vi "Main.vi"() -> ()   [LabVIEW 2021]
uses:
  Sub VIs/Trajectory Control/Trajectory_Control.ctl
  Sub VIs/Logging/Controller Data.ctl
  Sub VIs/Drive Motor/Drive Motor Data.ctl
  Sub VIs/Steering Motor/Steering Motor Data.ctl
  Sub VIs/State Estimator/State Estimate.ctl
  Sub VIs/State Estimator/Measurements.ctl
  Sub VIs/IMU/IMU Data.ctl
  Sub VIs/Steering Motor Encoder/Steering Motor Encoder Data.ctl
  Sub VIs/GNSS/GNSS Data.ctl
  <vilib>/Utility/RT CPU Load.ctl
  Sub VIs/Logging/Log Level.ctl
  <vilib>/Platform/TimedLoop/XDataNode/timing_clust.ctl
  <vilib>/Platform/TimedLoop/XDataNode/nitl_modes.ctl
  <vilib>/Platform/TimedLoop/XDataNode/wakeup.ctl
  Sub VIs/Steering Motor/Steering Motor Handle.ctl
  <vilib>/platform/TimedLoop/XDataNode/XDataNode.xnode
  <vilib>/Platform/TimedLoop/XDataNode/XDNodeRunTimeDep.lvlib
  <vilib>/NI_Real-Time Target Support.lvlib
panel:
  in  "Set Speed / Set Current\n(Built-in)  /  (PI Controller)":bool
  in  "Current at Steady State":dbl=5.5
  in  "Threshold":dbl=0.5
  out "?":bool
  in  "Open Loop Current Flag":bool
  in  "Open Loop Current":dbl min=0.0
  out "Abort Trajectory Enabled":bool
  out "Roll angle (rad)":dbl(graph)
  out "Indoor Enabled 2":bool
  in  "Indoor (RollRef)":bool
  out "Indoor Enabled":bool
  in  "Indoor (NoGPS)":bool
  out "Input and Motor Current (A)":T1(graph)
  out "Gyroscope (rad/s)":T2(graph)
  in  "No Kf":bool
  out "No Kf flag":bool
  in  "Kf":dbl
  in  "Abort Trajectory":bool
  in  "Kp":dbl
  in  "Ki":dbl
  out "Speed":bool
  in  "?":bool
  out "RPM":bool
  in  "Drive Motor Ref Speed (m/s)":dbl
  in  "file path (trajectorymat)":path=path "c:/ni-rt/startup/trajectorymat_parking_line.csv"
  in  "file path (matrixmat)":path=path "c:/ni-rt/startup/matrixmat_default.csv"
  out "velocity":dbl(graph)
  out "CPU loads":T3[](array[typedef]) {"ISR (%)" format="%#.2f"; "Idle (%)" format="%#.2f"; "Background (%)" format="%#.2f"; "Normal (%)" format="%#.2f"; "Above Normal (%)" format="%#.2f"; "High (%)" format="%#.2g"; "Timed Structures (%)" format="%#.2g"; "Time Critical (%)" format="%#.2g"; "Total (%)" format="%#.2g"}
  out "Measurements (Debug)":T4 {"GNSS Data"."Longitude (deg)" format="%#.10g"; "GNSS Data"."Latitude (deg)" format="%#.10g"; "GNSS Data"."Longitude (rad)" format="%#_10g"; "GNSS Data"."Latitude (rad)" format="%#_10g"}
  out "State Estimate (Debug)":T8 {"Y (m)" format="%#_10g"; "X (m)" format="%#_10g"}
  out "Motor Controllers (Debug)":T9
  out "Trajectory (Debug)":T12
  out "State estimator Ts check":bool
  out "E2 limit hit":bool
  out "E1 limit hit":bool
  out "XY trajectory (0 is bikeposition)":T13(graph)
  out "Y-Offset":dbl
  out "X-Offset":dbl
  in  "Reset and Init trajectory":bool
  in  "Drive Motor Ref Angular Speed (rad/s)":dbl
  in  "Enable Steering Motor":bool
  out "Steering Motor Enabled":bool
  out "Abort":bool
  in  "Reset Steering Motor Encoder":bool
  in  "Stop Button":bool
  # "To be set before running"
  # "PI Speed Controller"
  # "Scooter: \nKi=0.1, Kp=0.3\nGreen bike:\nKi=0.5, Kp=1.4\nRed bike\nKi=0.2, Kp=1.5"
  # "RED bike roller: 2.5\nGREEN bike roller: 5.5\nGREEN bike outside: 4.4"
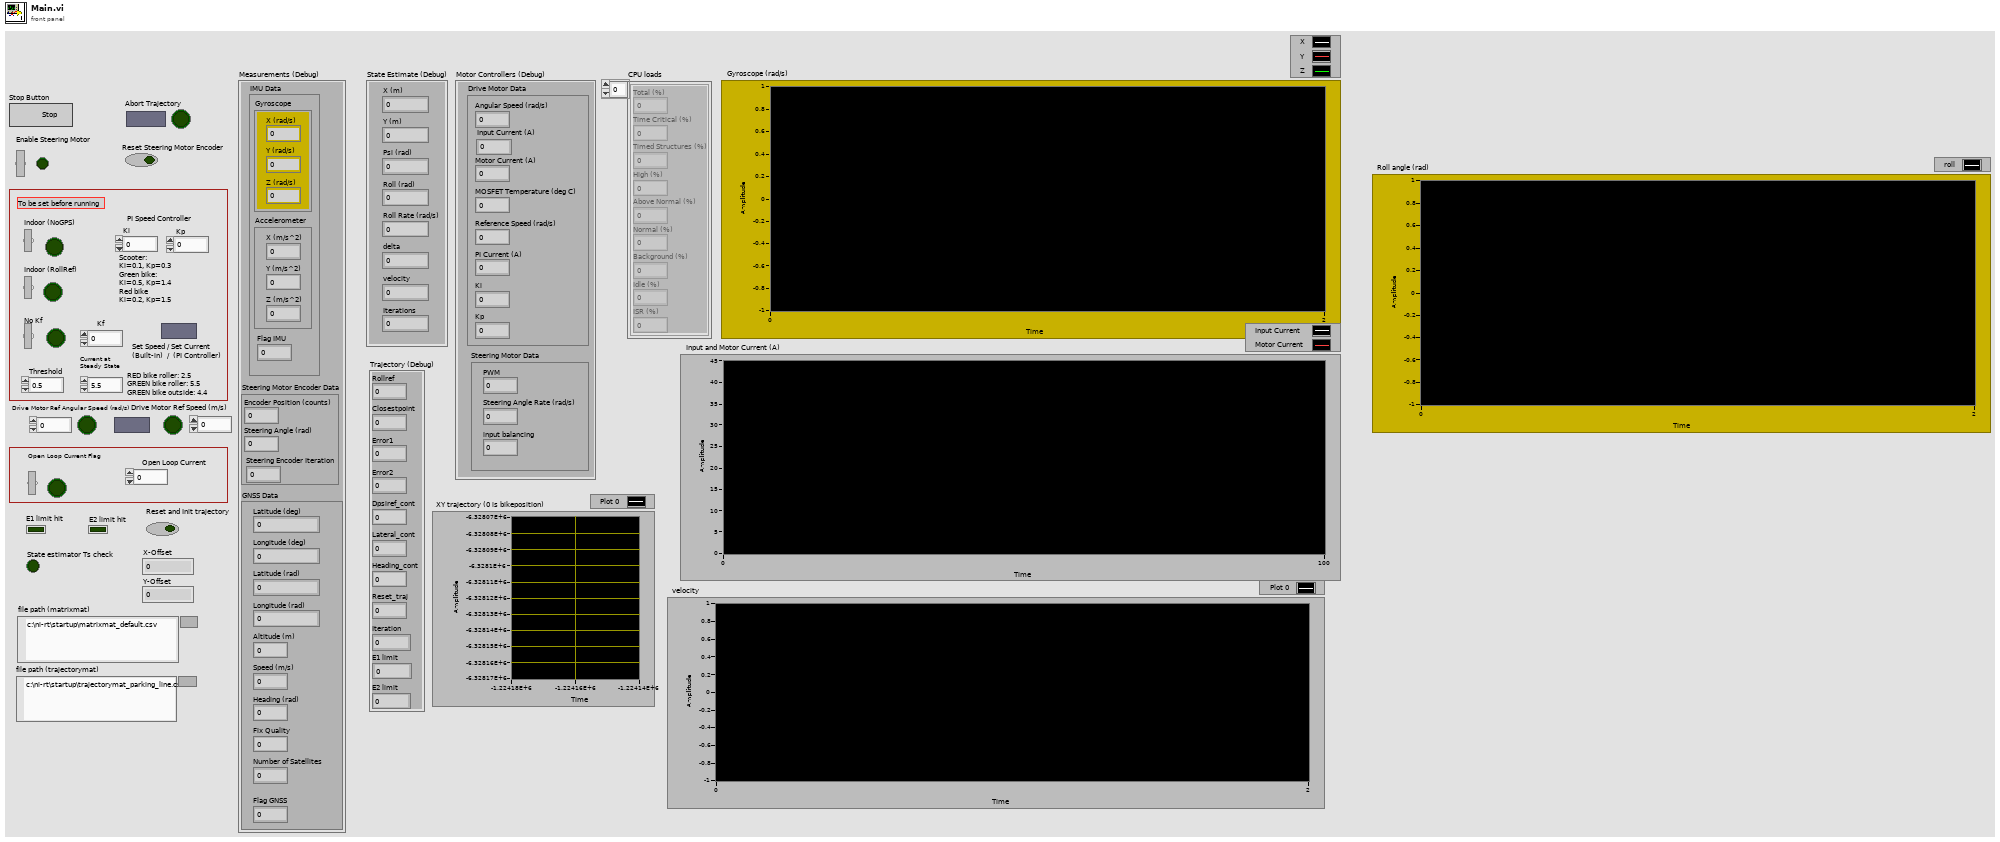
[diagram p1: front panel]
types:
  T1 = cluster{"Input Current (A)":dbl, "Motor Current (A)":dbl}
  T2 = cluster{"X (rad/s)":dbl, "Y (rad/s)":dbl, "Z (rad/s)":dbl}
  T3 = typedef "NI_Real-Time Target Support.lvlib/RT CPU Load.ctl" = cluster{"Total (%)":dbl, "Time Critical (%)":dbl, "Timed Structures (%)":dbl, "High (%)":dbl, "Above Normal (%)":dbl, "Normal (%)":dbl, "Background (%)":dbl, "Idle (%)":dbl, "ISR (%)":dbl}
  T4 = typedef "Measurements.ctl" = cluster{"IMU Data":T5, "Steering Motor Encoder Data":T6, "GNSS Data":T7}
  T5 = typedef "IMU Data.ctl" = cluster{"Gyroscope":cluster{"X (rad/s)":dbl, "Y (rad/s)":dbl, "Z (rad/s)":dbl}, "Accelerometer":cluster{"X (m/s^2)":dbl, "Y (m/s^2)":dbl, "Z (m/s^2)":dbl}, "Flag IMU":dbl}
  T6 = typedef "Steering Motor Encoder Data.ctl" = cluster{"Encoder Position (counts)":i32, "Steering Angle (rad)":dbl, "Steering Encoder Iteration":dbl}
  T7 = typedef "GNSS Data.ctl" = cluster{"Latitude (rad)":dbl, "Longitude (rad)":dbl, "Altitude (m)":dbl, "Speed (m/s)":dbl, "Heading (rad)":dbl, "Fix Quality":i32, "Number of Satellites":i32, "Latitude (deg)":dbl, "Longitude (deg)":dbl, "Flag GNSS":dbl}
  T8 = typedef "State Estimate.ctl" = cluster{"X (m)":dbl, "Y (m)":dbl, "Psi (rad)":dbl, "Roll (rad)":dbl, "Roll Rate (rad/s)":dbl, "delta":dbl, "velocity":dbl, "Iterations":dbl}
  T9 = typedef "Controller Data.ctl" = cluster{"Drive Motor Data":T10, "Steering Motor Data":T11}
  T10 = typedef "Drive Motor Data.ctl" = cluster{"Angular Speed (rad/s)":dbl, "Input Current (A)":dbl, "Motor Current (A)":dbl, "MOSFET Temperature (deg C)":dbl, "Reference Speed (rad/s)":dbl, "PI Current (A)":dbl, "Ki":dbl, "Kp":dbl}
  T11 = typedef "Steering Motor Data.ctl" = cluster{"PWM":dbl, "Steering Angle Rate (rad/s)":dbl, "input balancing":dbl}
  T12 = typedef "Trajectory_Control.ctl" = cluster{"Rollref":dbl, "Closestpoint":dbl, "Error1":dbl, "Error2":dbl, "Dpsiref_cont":dbl, "Lateral_cont":dbl, "Heading_cont":dbl, "Reset_traj":dbl, "Iteration":dbl, "E1 limit":u32, "E2 limit":u32}
  T13 = cluster{"Trajectory(X/Y/PSI)":dbl[], "Trajectory(X/Y/PSI)":dbl[]}
  T14 = cluster{"Steering Angle Rate":dbl, "rollReference":dbl, "roll":dbl, "rollRate":dbl, "Kp":dbl, "Kd":dbl, "steering_flag":i32}
  T15 = typedef "XDNodeRunTimeDep.lvlib/timing_clust.ctl" = cluster{"Expected End [f-1]":u64, "Actual End [f-1]":u64, "Finished Late? [f-1]":bool, "Expected End [i-1]":u64, "Actual End [i-1]":u64, "Finished Late? [i-1]":bool, "Expected Start [i]":u64, "Actual Start [i]":u64, "Expected Start [f]":u64, "Actual Start [f]":u64, "Source Name":string, "Structure Name":string, "Period":i64, "Deadline":i64, "Offset":i64, "Start":i64, "Priority":i32, "Timeout":i32, "Mode":T16, "Wakeup Reason":T17, "Error":errorcluster, "Source Type":string, "Secondary Source Type":string, "Global End Time":u64, "Global Start Time":u64, "Frame Duration":u64, "Iteration Duration":u64, "Assigned CPU":i32, "I/O Scan Engine Mode":u32}
  T16 = typedef "XDNodeRunTimeDep.lvlib/nitl_modes.ctl" = enum32{"No Change", "Process missed periods, maintain original phase", "Discard missed periods, maintain original phase", "Process missed periods, ignore original phase", "Discard missed periods, ignore original phase"}
  T17 = typedef "XDNodeRunTimeDep.lvlib/wakeup.ctl" = enum32{"Normal", "Aborted", "Asynchronous wakeup", "Timing source error", "Timed loop error", "Timeout"}
  T18 = typedef "Steering Motor Handle.ctl" = cluster{"Dummy":dbl}
  T19 = typedef "Log Level.ctl" = enum16{"Error", "Warning", "Info"}
  T20 = cluster{"B":dbl[], "A":dbl[][], "C":dbl[][], "D":dbl[], "K":dbl[][], "Trajectory":dbl[][], "Init":dbl[], "parameter":dbl[][], "K_noGPS":dbl[][]}
  T21 = typedef "Configuration.ctl" = cluster{"Accelerometer Bias":cluster{"X (m/s)":dbl, "Y (m/s)":dbl, "Z (m/s)":dbl}, "Gyroscope Bias":cluster{"X (m/s)":dbl, "Y (m/s)":dbl, "Z (m/s)":dbl}, "Steering Motor Gear Ratio":dbl, "Steering Pully Gear Ratio":dbl, "Steering Encoder CPR":dbl, "Steering Motor Max RPM":dbl, "Wheelbase (m)":dbl, "Fork Angle (rad)":dbl, "Balancing Controller":cluster{"Kp (/s)":dbl, "Kd (1)":dbl}, "Max Allowed Steering Angle (rad)":dbl, "Task Periods":cluster{"Emergency Stop (us)":i64, "IMU (us)":i64, "Steering Motor Encoder (us)":i64, "State Estimator (us)":i64, "Balancing Controller (us)":i64, "GNSS (us)":i64, "Logging (us)":i64, "Drive Motor (us)":i64, "Visualization (us)":i64}, "Drive Motor Gear Ratio":dbl, "lr":dbl, "lf":dbl, "lambda":dbl, "k1":dbl, "k2":dbl, "e1_max":dbl, "Ad_t":dbl, "Bd_t":dbl, "C_t":dbl, "D_t":dbl, "Wheel radius":dbl}
  T22 = typedef "NI_Matrix.lvlib/RealMatrix.ctl" = dbl[][]
  T23 = typedef "GNSS Handle.ctl" = cluster{"VISA Resource Name":refnum<visa-resource-name>}
  T24 = typedef "IMU Handle.ctl" = cluster{"I2C address":u8}
  T25 = typedef "Drive Motor Handle.ctl" = cluster{"VISA Resource Name":refnum<visa-resource-name>}
  T26 = typedef "Log Handle.ctl" = cluster{"Data File":refnum<file>, "Event File":refnum<file>}
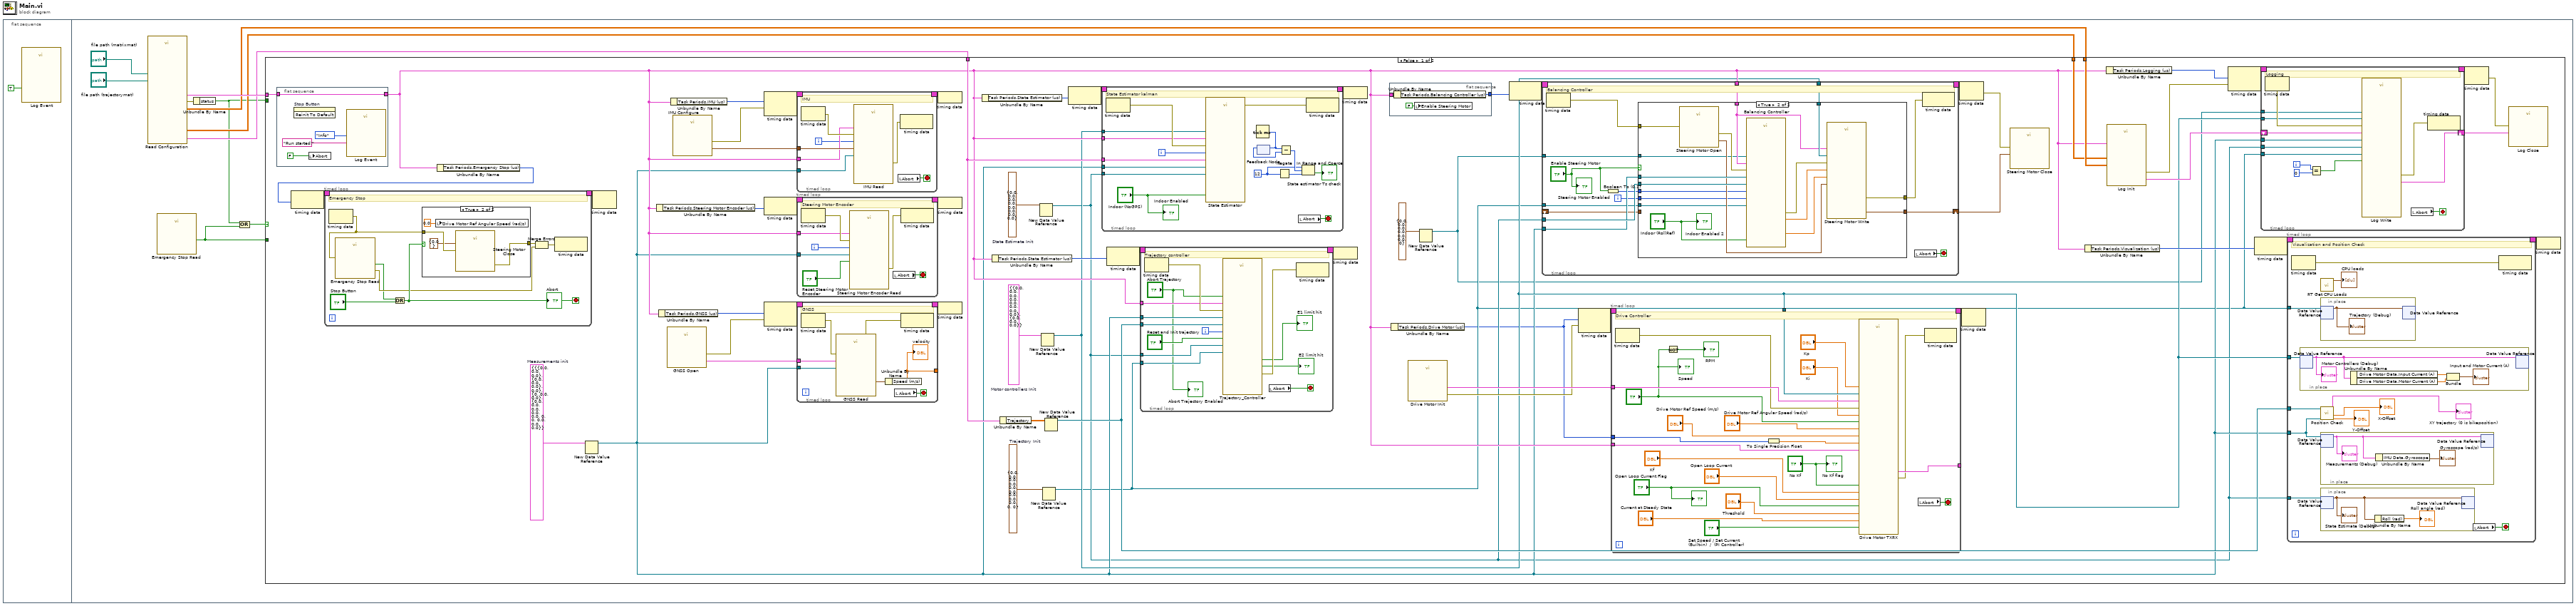
[diagram p0: block diagram]
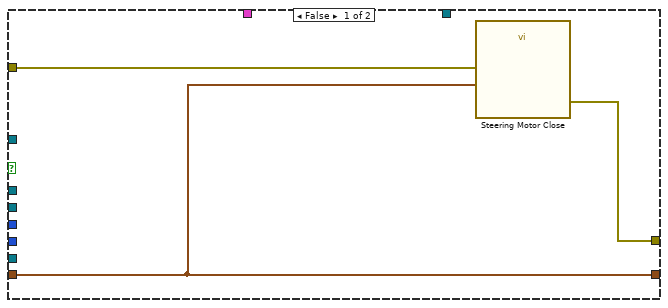
[diagram p2: hidden frame]
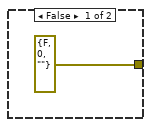
[diagram p3: hidden frame]
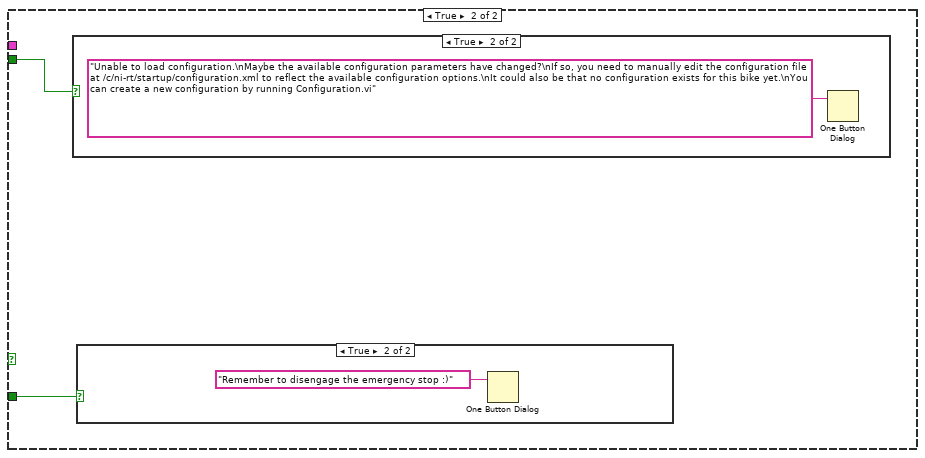
[diagram p4: hidden frame]
diagram:
  n1 = flat-sequence {
    frame #0 {
      n2 = call "Log Event.vi"("Clear Log"=TRUE) -> ()  [unwired: 10 in, 1 out]
    }
    frame #1 {
      n3 = call "Read Configuration.vi"("file path (trajectorymat)"="file path (trajectorymat)", "file path (matrixmat)"="file path (matrixmat)") -> ("values loded in xml files"=w9:T20, "configuration"=w11:T21, "value"=w6:T22, "error out"=w10:errorcluster, "Init trajectory (2)"=w8:dbl[][])  [unwired: 3 in, 2 out]
      n4 = call "Emergency Stop Read.vi"() -> ("Emergency Stop"=w2:bool)  [unwired: 10 in, 1 out]
      n5 = Unbundle By Name(w10) -> ("status"=w3:bool)
      n6 = Compound Arithmetic op=OR(w3, w2) -> (w7:bool)
      n7 = case shown="False" w7 {
        tunnel: w3 -> [_ w326]
        tunnel: w11 -> [w49 _]
        tunnel: w9 -> [w25 _]
        tunnel: w2 -> [_ w325]
        tunnel: w8 -> [w41 _]
        tunnel: w6 -> [w27 _]
        frame False {
          w33 = T12 {"Rollref"=0.0, "Closestpoint"=0.0, "Error1"=0.0, "Error2"=0.0, "Dpsiref_cont"=0.0, "Lateral_cont"=0.0, "Heading_cont"=0.0, "Reset_traj"=0.0, "Iteration"=0.0, "E1 limit"=0, "E2 limit"=0}  # Trajectory Init
          w42 = T8 {"X (m)"=0.0, "Y (m)"=0.0, "Psi (rad)"=0.0, "Roll (rad)"=0.0, "Roll Rate (rad/s)"=0.0, "delta"=0.0, "velocity"=0.0, "Iterations"=0.0}  # State Estimate Init
          w48 = T9 {"Drive Motor Data"={"Angular Speed (rad/s)"=0.0, "Input Current (A)"=0.0, "Motor Current (A)"=0.0, "MOSFET Temperature (deg C)"=0.0, "Reference Speed (rad/s)"=0.0, "PI Current (A)"=0.0, "Ki"=0.0, "Kp"=0.0}, "Steering Motor Data"={"PWM"=0.0, "Steering Angle Rate (rad/s)"=0.0, "input balancing"=0.0}}  # Motor controllers Init
          w70 = T4 {"IMU Data"={"Gyroscope"={"X (rad/s)"=0.0, "Y (rad/s)"=0.0, "Z (rad/s)"=0.0}, "Accelerometer"={"X (m/s^2)"=0.0, "Y (m/s^2)"=0.0, "Z (m/s^2)"=0.0}, "Flag IMU"=0.0}, "Steering Motor Encoder Data"={"Encoder Position (counts)"=0, "Steering Angle (rad)"=0.0, "Steering Encoder Iteration"=0.0}, "GNSS Data"={"Latitude (rad)"=0.0, "Longitude (rad)"=0.0, "Altitude (m)"=0.0, "Speed (m/s)"=0.0, "Heading (rad)"=0.0, "Fix Quality"=0, "Number of Satellites"=0, "Latitude (deg)"=0.0, "Longitude (deg)"=0.0, "Flag GNSS"=0.0}}  # Measurements init
          n8 = flat-sequence {
            tunnel: [w322] -> w24
            tunnel: w49 -> [w322]
            frame #0 {
              n9 = invoke on="Stop Button" class="Bool (strict)" method="Reinit To Default"() -> ()  [unwired: 3 in, 3 out]
              n10 = local write "Abort"(FALSE ("Abort")) -> ()
              n11 = call "Log Event.vi"("Message"="Run started!", "Log Level"=Log_Level."Info") -> ()  [unwired: 9 in, 1 out]
            }
          }
          n12 = Unbundle By Name(w24) -> ("Task Periods.Emergency Stop (us)"=w12:i64)
          n13 = node-c288(w12) -> (w69:T15)
          n14 = timed-loop {
            timing: w69 -> [_]
            timing-out: [_] -> w68
            stop <- w304 stop-if-true
            # "Emergency Stop"
            n15 = node-c288() -> (w306:errorcluster)  [unwired: 1 in]
            n16 = call "Emergency Stop Read.vi"("Error In"=w306) -> ("Emergency Stop"=w301:bool, "Error Out"=w302:errorcluster)  [unwired: 9 in]
            n17 = Or(x=w301, y="Stop Button") -> (x .or. y?=w304:bool)
            "Abort" <- w304
            n18 = case shown="True" w304 {
              tunnel: w306 -> [_ w311]
              tunnel: [errorcluster {"status"=FALSE, "code"=0, "source"=""} ("Error Out") w310] -> w303
              frame False {
              }
              frame True {
                n19 = local write "Drive Motor Ref Angular Speed (rad/s)"(0.0 ("Drive Motor Angular Speed (rad/s)")) -> ()
                n20 = call "Steering Motor Close.vi"("Steering Motor Handle"=T18 {"Dummy"=0.0}, "Error In"=w311) -> ("Error Out"=w310:errorcluster)  [unwired: 9 in]
              }
            }
            n21 = Merge Errors(w303, w302) -> (w305:errorcluster)
            n22 = node-c288(w305) -> ()  [unwired: 1 out]
          }
          n23 = New Data Value Reference(data value=w70) -> (data value reference=w20:refnum<data-value>)  [unwired: 1 in, 1 out]
          n24 = node-c288(w68) -> ()  [unwired: 1 out]
          n25 = Unbundle By Name(w24) -> ("Task Periods.Steering Motor Encoder (us)"=w54:i64)
          n26 = Unbundle By Name(w24) -> ("Task Periods.GNSS (us)"=w51:i64)
          n27 = call "GNSS Open.vi"() -> ("GNSS Handle"=w52:T23, "Error Out"=w53:errorcluster)  [unwired: 10 in]
          n28 = Unbundle By Name(w24) -> ("Task Periods.IMU (us)"=w55:i64)
          n29 = call "IMU Configure.vi"() -> ("IMU Handle"=w56:T24, "Error Out"=w57:errorcluster)  [unwired: 10 in]
          n30 = node-c288(w55, w57) -> (w63:T15)
          n31 = node-c288(w54) -> (w61:T15)
          n32 = node-c288(w51, w53) -> (w59:T15)
          n33 = timed-loop {
            timing: w63 -> [_]
            timing-out: [_] -> w62
            tunnel: w56 -> [w240]
            tunnel: w20 -> [w238]
            tunnel: w24 -> [w237]
            i -> [w236]
            stop <- w239 stop-if-true
            # "IMU"
            n34 = node-c288() -> (w242:errorcluster)  [unwired: 1 in]
            n35 = call "IMU Read.vi"("Configuration"=w237, "Measurement In"=w238, "Flag IMU"=w236, "IMU Handle"=w240, "Error In"=w242) -> ("Error Out"=w241:errorcluster)  [unwired: 4 in, 2 out]
            n36 = local read "Abort"() -> (w239:bool)
            n37 = node-c288(w241) -> ()  [unwired: 1 out]
          }
          n38 = timed-loop {
            timing: w61 -> [_]
            timing-out: [_] -> w60
            tunnel: w20 -> [w222]
            tunnel: w24 -> [w220]
            i -> [w221]
            stop <- w223 stop-if-true
            # "Steering Motor Encoder"
            n39 = node-c288() -> (w226:errorcluster)  [unwired: 1 in]
            n40 = call "Steering Motor Encoder Read.vi"("Configuration"=w220, "Measurement In"=w222, "Flag Steering Encoder"=w221, "Reset Counter"="Reset Steering Motor Encoder", "Error In"=w226) -> ("Error Out"=w225:errorcluster)  [unwired: 4 in, 2 out]
            n41 = local read "Abort"() -> (w223:bool)
            n42 = node-c288(w225) -> ()  [unwired: 1 out]
          }
          n43 = timed-loop {
            timing: w59 -> [_]
            timing-out: [_] -> w58
            tunnel: w52 -> [w209]
            tunnel: w20 -> [w205]
            tunnel: [w203] -> _
            stop <- w206 stop-if-true
            # "GNSS"
            n44 = node-c288() -> (w208:errorcluster)  [unwired: 1 in]
            n45 = call "GNSS Read.vi"("Measurement In"=w205, "GNSS Handle"=w209, "Error In"=w208) -> ("GNSS Data"=w204:T7, "Error Out"=w207:errorcluster)  [unwired: 6 in, 1 out]
            n46 = Unbundle By Name(w204) -> ("Speed (m/s)"=w203:dbl)
            "velocity" <- w203
            n47 = local read "Abort"() -> (w206:bool)
            n48 = node-c288(w207) -> ()  [unwired: 1 out]
          }
          n49 = node-c288(w62) -> ()
          n50 = node-c288(w60) -> ()
          n51 = node-c288(w58) -> ()
          n52 = Unbundle By Name(w24) -> ("Task Periods.State Estimator (us)"=w22:i64)
          n53 = Unbundle By Name(w24) -> ("Task Periods.State Estimator (us)"=w34:i64)
          n54 = Unbundle By Name(w25) -> ("Trajectory"=w32:dbl[][])
          n55 = New Data Value Reference(data value=w42) -> (data value reference=w19:refnum<data-value>)  [unwired: 1 in, 1 out]
          n56 = New Data Value Reference(data value=w48) -> (data value reference=w21:refnum<data-value>)  [unwired: 1 in, 1 out]
          n57 = New Data Value Reference(data value=w33) -> (data value reference=w18:refnum<data-value>)  [unwired: 1 in, 1 out]
          n58 = New Data Value Reference(data value=w32) -> (data value reference=w26:refnum<data-value>)  [unwired: 1 in, 1 out]
          n59 = node-c288(w22) -> (w36:T15)
          n60 = timed-loop {
            timing: w36 -> [_]
            timing-out: [_] -> w35
            tunnel: w20 -> [w131]
            tunnel: w25 -> [w134]
            tunnel: w21 -> [w130]
            tunnel: w19 -> [w129]
            tunnel: w24 -> [w133]
            i -> [w132]
            stop <- w137 stop-if-true
            w123 = i64 12 ("y")
            # "State Estimator kalman"
            n61 = node-c288() -> (w136:errorcluster)  [unwired: 1 in]
            n62 = call "State Estimator.vi"("Error In"=w136, "State Estimate In"=w129, "Matrix"=w134, "Configuration"=w133, "Iteration"=w132, "Measurement In"=w131, "Balancing controller In"=w130, "Indoor&NoGPS"="Indoor (NoGPS)") -> ("Error out"=w135:errorcluster)  [unwired: 6 in, 1 out]
            n63 = Tick Count (ms)() -> (millisecond timer value=w128:u32)
            n64 = feedback-in #1(w128) -> ()
            n65 = feedback #1() -> (w127:u32)  [unwired: 1 in]
            n66 = Negate(x=w123) -> (-x=w124:i64)
            n67 = Subtract(x=w128, y=w127) -> (x-y=w125:u32)
            n68 = local read "Abort"() -> (w137:bool)
            n69 = In Range and Coerce(upper limit=w123, x=w125, lower limit=w124) -> (In Range?=→"State estimator Ts check":bool)  [unwired: 1 out]
            n70 = node-c288(w135) -> ()  [unwired: 1 out]
            "Indoor Enabled" <- "Indoor (NoGPS)"
          }
          n71 = node-c288(w34) -> (w14:T15)
          n72 = timed-loop {
            timing: w14 -> [_]
            timing-out: [_] -> w13
            tunnel: w19 -> [w82]
            tunnel: w24 -> [w79]
            tunnel: w20 -> [w77]
            tunnel: w26 -> [w76]
            tunnel: w18 -> [w74]
            i -> [w78]
            stop <- w83 stop-if-true
            # "Trajectory controller"
            n73 = node-c288() -> (w80:errorcluster)  [unwired: 1 in]
            n74 = call "Trajectory_Controller.vi"("Error In"=w80, "reset"=w78, "Abort Trajectory"="Abort Trajectory", "Configuration"=w79, "State Estimate In"=w82, "Reset and Init trajectory"="Reset and Init trajectory", "RefTraj in"=w76, "Trajectory In"=w74, "Measurement In"=w77) -> ("Error out"=w81:errorcluster, "E1 limit"=→"E1 limit hit":bool, "E2 limit"=→"E2 limit hit":bool)  [unwired: 2 in, 2 out]
            n75 = local read "Abort"() -> (w83:bool)
            n76 = node-c288(w81) -> ()  [unwired: 1 out]
            "Abort Trajectory Enabled" <- "Abort Trajectory"
          }
          n77 = node-c288(w13) -> ()
          n78 = node-c288(w35) -> ()
          n79 = flat-sequence {
            tunnel: [w254] -> w50
            tunnel: w24 -> [w253]
            frame #0 {
              n80 = Unbundle By Name(w253) -> ("Task Periods.Balancing Controller (us)"=w254:i64)
              n81 = local write "Enable Steering Motor"(FALSE ("Enable Steering Motor")) -> ()
            }
          }
          n82 = Unbundle By Name(w24) -> ("Task Periods.Drive Motor (us)"=w15:i64)
          n83 = call "Drive Motor Init.vi"() -> ("Drive Motor Handle"=w38:T25, "Error Out"=w37:errorcluster)  [unwired: 10 in]
          n84 = New Data Value Reference(data value=T14 {"Steering Angle Rate"=0.0, "rollReference"=0.0, "roll"=0.0, "rollRate"=0.0, "Kp"=0.0, "Kd"=0.0, "steering_flag"=0} ("output cluster")) -> (data value reference=w16:refnum<data-value>)  [unwired: 1 in, 1 out]
          n85 = node-c288(w50) -> (w67:T15)
          n86 = timed-loop {
            timing: w67 -> [_]
            timing-out: [_] -> w66
            tunnel: w19 -> [w265]
            tunnel: w20 -> [w264]
            shift-right: [w266] -> w65
            shift-left: _ -> [w263]
            tunnel: w24 -> [w262]
            tunnel: w21 -> [w261]
            tunnel: w18 -> [w260]
            tunnel: w16 -> [w257]
            i -> [w256]
            stop <- w269 stop-if-true
            # "Balancing Controller"
            n87 = node-c288() -> (w268:errorcluster)  [unwired: 1 in]
            n88 = Boolean To (0,1)(Boolean="Enable Steering Motor") -> (0, 1=w258:i16)
            n89 = case shown="True" "Enable Steering Motor" {
              tunnel: w268 -> [w272 w283]
              tunnel: [w271 w288] -> w267
              tunnel: [w270 w287] -> w266
              tunnel: w265 -> [_ w285]
              tunnel: w264 -> [_ w284]
              tunnel: w263 -> [w270 _]
              tunnel: w262 -> [_ w279]
              tunnel: w261 -> [_ w280]
              tunnel: w260 -> [_ w278]
              tunnel: w258 -> [_ w276]
              tunnel: w257 -> [_ w275]
              tunnel: w256 -> [_ w274]
              frame False {
                n90 = call "Steering Motor Close.vi"("Steering Motor Handle"=w270, "Error In"=w272) -> ("Error Out"=w271:errorcluster)  [unwired: 9 in]
              }
              frame True {
                n91 = call "Steering Motor Open.vi"("Error In"=w283) -> ("Steering Motor Handle"=w281:T18, "Error Out"=w282:errorcluster)  [unwired: 9 in]
                n92 = call "Balancing Controller.vi"("Error In"=w282, "steering indicator flag"=w276, "Trajectory In"=w278, "Balance In"=w275, "State Estimate In"=w285, "t"=w274, "Measurement In"=w284, "Indoor (RollRef)"="Indoor (RollRef)", "Configuration"=w279) -> ("Input balancing"=w277:dbl, "Error Out"=w289:errorcluster, "Steering Angle Rate (rad/s)"=w286:dbl)  [unwired: 3 in, 1 out]
                n93 = call "Steering Motor Write.vi"("Configuration"=w279, "Input balancing"=w277, "Controller Data In"=w280, "Steering Angle Rate (rad/s)"=w286, "Steering Motor Handle In"=w281, "Error In"=w289) -> ("Steering Motor Handle Out"=w287:T18, "Error Out"=w288:errorcluster)  [unwired: 2 in, 2 out]
                "Indoor Enabled 2" <- "Indoor (RollRef)"
              }
            }
            n94 = local read "Abort"() -> (w269:bool)
            n95 = node-c288(w267) -> ()  [unwired: 1 out]
            "Steering Motor Enabled" <- "Enable Steering Motor"
          }
          n96 = node-c288(w15, w37) -> (w40:T15)
          n97 = timed-loop {
            timing: w40 -> [_]
            timing-out: [_] -> w39
            tunnel: w38 -> [w166]
            tunnel: w24 -> [w162]
            tunnel: w21 -> [w163]
            tunnel: [w167] -> _
            tunnel: w15 -> [w154]
            stop <- w168 stop-if-true
            # "Drive Controller"
            n98 = node-c288() -> (w165:errorcluster)  [unwired: 1 in]
            n99 = Not(x="?") -> (.not. x?=→"RPM":bool)
            n100 = To Single Precision Float(number=w154) -> (single precision float=w155:sgl)
            n101 = call "Drive Motor TXRX.vi"("Error In"=w165, "Drive Motor Handle In"=w166, "Open Loop Current Flag"="Open Loop Current Flag", "Tasking Period"=w155, "RPM Control (rad/s)"="Drive Motor Ref Angular Speed (rad/s)", "Controller Data In"=w163, "Speed Control (m/s)"="Drive Motor Ref Speed (m/s)", 9:w162, "Set Current / Set RPM"="Set Speed / Set Current\n(Built-in)  /  (PI Controller)", "Threshold"="Threshold", "Current at Steady State"="Current at Steady State", "No Kf"="No Kf", "Ki"="Ki", "RPM / Speed"="?", "Kp"="Kp", "Open Loop Current"="Open Loop Current", "Kf"="Kf") -> ("Error Out"=w164:errorcluster, "Drive Motor Handle Out"=w167:T25)  [unwired: 7 in, 2 out]
            n102 = local read "Abort"() -> (w168:bool)
            n103 = node-c288(w164) -> ()  [unwired: 1 out]
            "Speed" <- "?"
            "No Kf flag" <- "No Kf"
            "?" <- "Open Loop Current Flag"
          }
          n104 = node-c288(w66) -> (w64:errorcluster)
          n105 = node-c288(w39) -> ()  [unwired: 1 out]
          n106 = call "Steering Motor Close.vi"("Steering Motor Handle"=w65, "Error In"=w64) -> ()  [unwired: 9 in, 1 out]
          n107 = Unbundle By Name(w24) -> ("Task Periods.Visualization (us)"=w28:i64)
          n108 = Unbundle By Name(w24) -> ("Task Periods.Logging (us)"=w23:i64)
          n109 = call "Log Init.vi"("Configuration"=w24, "Matrices"=w27, "Trajectory"=w41) -> ("Log Handle"=w43:T26, "Error Out"=w45:errorcluster)  [unwired: 7 in]
          n110 = node-c288(w23, w45) -> (w47:T15)
          n111 = node-c288(w28) -> (w30:T15)
          n112 = timed-loop {
            timing: w47 -> [_]
            timing-out: [_] -> w46
            tunnel: w20 -> [w181]
            tunnel: w19 -> [w184]
            shift-right: [w186] -> w31
            shift-left: w43 -> [w185]
            tunnel: w21 -> [w183]
            tunnel: w18 -> [w182]
            tunnel: w16 -> [w179]
            i -> [w180]
            stop <- w191 stop-if-true
            # "Logging"
            n113 = node-c288() -> (w188:errorcluster)  [unwired: 1 in]
            n114 = Equal?(x=w180, y=0) -> (x = y?=w189:bool)
            n115 = call "Log Write.vi"("Error In"=w188, "Write Header"=w189, "Log Handle In"=w185, "Trajectory In"=w182, "State Estimate In"=w184, "Measurement In"=w181, "Controller Data In"=w183, "Balance In"=w179) -> ("Error Out"=w187:errorcluster, "Log Handle Out"=w186:T26)  [unwired: 1 in, 5 out]
            n116 = local read "Abort"() -> (w191:bool)
            n117 = node-c288(w187) -> ()  [unwired: 1 out]
          }
          n118 = timed-loop {
            timing: w30 -> [_]
            timing-out: [_] -> w29
            tunnel: w26 -> [w102]
            tunnel: w20 -> [w93]
            tunnel: w21 -> [w98]
            tunnel: w19 -> [w97]
            tunnel: w18 -> [w96]
            stop <- w94 stop-if-true
            # "Visualization and Position Check"
            n119 = node-c288() -> (w103:errorcluster)  [unwired: 1 in]
            n120 = in-place {
              n121 = in-place-dvr #2(w98) -> (w108:T9)  [unwired: 1 out]
              "Motor Controllers (Debug)" <- w108
              n122 = Unbundle By Name(w108) -> ("Drive Motor Data.Input Current (A)"=w107:dbl, "Drive Motor Data.Motor Current (A)"=w106:dbl)
              n123 = Bundle("Input Current (A)"=w107, "Motor Current (A)"=w106) -> (→"Input and Motor Current (A)":T1)  [unwired: 1 in]
              n124 = in-place-dvr #2(w108) -> ()  [unwired: 2 out]
            }
            n125 = call <vilib>:"RT Get CPU Loads.vi"() -> ("CPU loads"=→"CPU loads":T3[])  [unwired: 10 in, 1 out]
            n126 = in-place {
              n127 = in-place-dvr #3(w96) -> (w104:T12)  [unwired: 1 out]
              "Trajectory (Debug)" <- w104
              n128 = in-place-dvr #3(w104) -> ()  [unwired: 2 out]
            }
            n129 = in-place {
              n130 = in-place-dvr #4(w93) -> (w112:T4)  [unwired: 1 out]
              "Measurements (Debug)" <- w112
              n131 = Unbundle By Name(w112) -> ("IMU Data.Gyroscope"=→"Gyroscope (rad/s)":T2)
              n132 = in-place-dvr #4(w112) -> ()  [unwired: 2 out]
            }
            n133 = in-place {
              n134 = in-place-dvr #5(w97) -> (w110:T8)  [unwired: 1 out]
              "State Estimate (Debug)" <- w110
              n135 = Unbundle By Name(w110) -> ("Roll (rad)"=→"Roll angle (rad)":dbl)
              n136 = in-place-dvr #5(w110) -> ()  [unwired: 2 out]
            }
            n137 = call "Position Check.vi"("data value reference 2"=w93, "data value reference"=w102) -> ("Y-Offset"=→"Y-Offset":dbl, "X-Offset"=→"X-Offset":dbl, "XY Graph"=→"XY trajectory (0 is bikeposition)":T13)  [unwired: 7 in]
            n138 = local read "Abort"() -> (w94:bool)
            n139 = node-c288(w103) -> ()  [unwired: 1 out]
          }
          n140 = node-c288(w46) -> (w44:errorcluster)
          n141 = call "Log Close.vi"("Log Handle In"=w31, "Error In"=w44) -> ()  [unwired: 9 in, 1 out]
          n142 = node-c288(w29) -> ()
        }
        frame True {
          n143 = case shown="True" w326 {
            frame False {
            }
            frame True {
              n144 = One Button Dialog(message="Unable to load configuration.\nMaybe the available configuration parameters have changed?\nIf so, you need to manually edit the configuration file at /c/ni-rt/startup/configuration.xml to reflect the available configuration options.\nIt could also be that no configuration exists for this bike yet.\nYou can create a new configuration by running Configuration.vi") -> ()  [unwired: 1 in, 1 out]
            }
          }
          n145 = case shown="True" w325 {
            frame False {
            }
            frame True {
              n146 = One Button Dialog(message="Remember to disengage the emergency stop :)") -> ()  [unwired: 1 in, 1 out]
            }
          }
        }
      }
    }
  }
